vi "Get Transmission Type.vi"(8 "error in":errorcluster, 11 "RPDO Communication Parameter in":refnum<class "RPDO Communication Parameter.lvclass">) -> (0 "error out":errorcluster, 2 "Transmission Type":u8(ring)=254 format="%.0x" items=["synchronous"=0, "synchronous"=240, "reserved"=241, "reserved"=253, "event-driven (manufacturer-specific)"=254, "event-driven (device profile and application profile specific)"=255], 3 "RPDO Communication Parameter out":refnum<class "RPDO Communication Parameter.lvclass">)   [LabVIEW 2020, in "CANopen.lvlib" / "RPDO Communication Parameter.lvclass"]
uses:
  RPDO Communication Parameter.lvclass
  RPDO Communication Parameter.lvclass/RPDO Communication Parameter.ctl
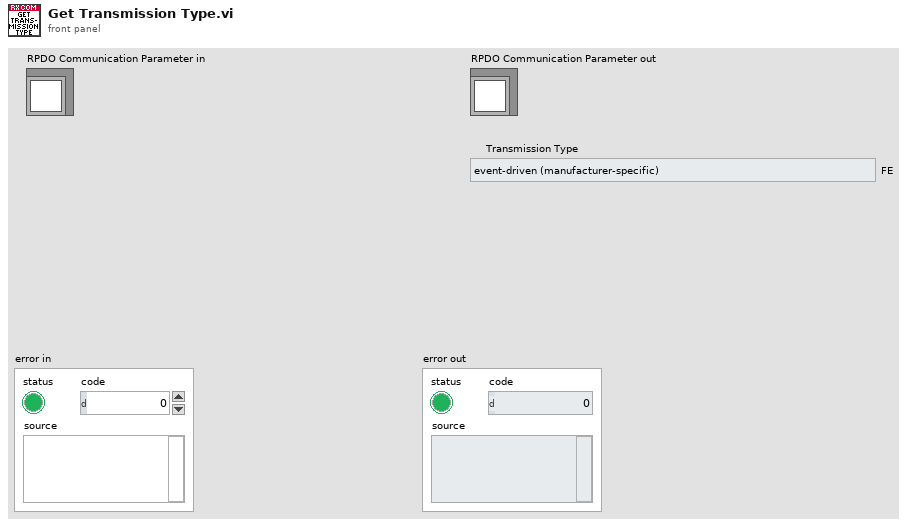
[diagram p1: front panel]
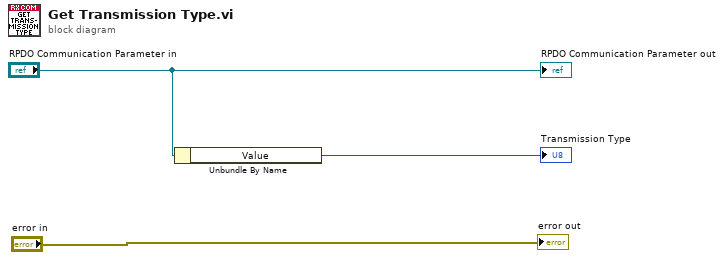
[diagram p0: block diagram]
diagram:
  n1 = Unbundle By Name("RPDO Communication Parameter in") -> ("Value"=→"Transmission Type":u8)
  "error out" <- "error in"
  "RPDO Communication Parameter out" <- "RPDO Communication Parameter in"
